vi "Database Queue Handler.vi"(7 "Action":T3, 8 "error in (no error)":errorcluster, 10 "Message in":T1, 11 "Queue in":refnum<queue>) -> (0 "error out":errorcluster, 2 "Message out":T1, 3 "Queue out":refnum<queue>)   [LabVIEW 2017]
uses:
  Type Definitions/Queue FG Options.ctl
  Type Definitions/Database Message.ctl
  Type Definitions/Database States.ctl
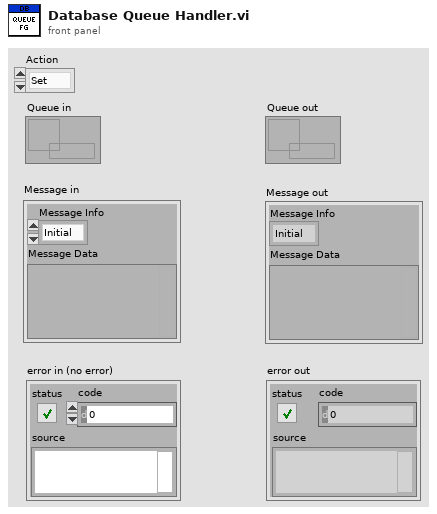
[diagram p1: front panel]
types:
  T1 = typedef "Database Message.ctl" = cluster{"Message Info":T2, "Message Data":variant}
  T2 = typedef "Database States.ctl" = enum16{"Initial", "Verify", "Balance Inquiry", "Deposit", "Withdrawal", "Terminate", "Shutdown"}
  T3 = typedef "Queue FG Options.ctl" = enum16{"Set", "Get", "Read", "Write"}
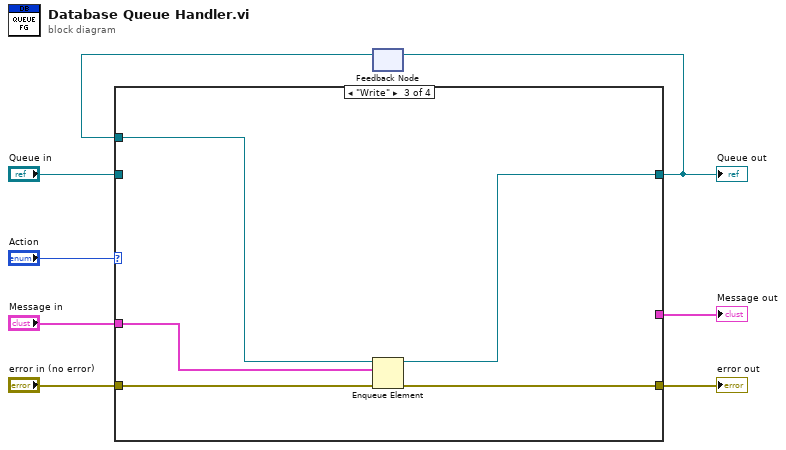
[diagram p0: block diagram]
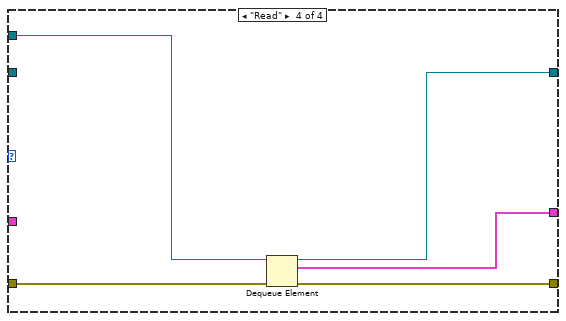
[diagram p4: hidden frame]
diagram:
  n1 = feedback #1() -> (w5:refnum<queue>)  [unwired: 1 in]
  n2 = case shown="\"Write\"" "Action" {
    tunnel: "error in (no error)" -> [w10 w12 w17 w22]
    tunnel: [w10 w12 w16 w21] -> w6
    tunnel: w5 -> [_ w11 w15 w20]
    tunnel: "Message in" -> [_ _ w14 _]
    tunnel: [w9 w11 w13 w19] -> w3
    tunnel: "Queue in" -> [w9 _ _ _]
    tunnel: [_ _ _ w18] -> w1
    frame "Set" {
    }
    frame "Get", Default {
    }
    frame "Write" {
      n3 = Enqueue Element(queue=w15, element=w14, error in (no error)=w17) -> (queue out=w13:refnum<queue>, error out=w16:errorcluster)  [unwired: 1 in, 1 out]
    }
    frame "Read" {
      n4 = Dequeue Element(queue=w20, error in (no error)=w22) -> (queue out=w19:refnum<queue>, element=w18:T1, error out=w21:errorcluster)  [unwired: 1 in, 1 out]
    }
  }
  "error out" <- w6
  "Message out" <- w1
  "Queue out" <- w3
  n5 = feedback-in #1(w3) -> ()
